vi "Teleop.vi"(10 "Match Info":T1={"Autonomous Elapsed Seconds"=0.0, "TeleOp Elapsed Seconds"=0.0, "Disabled Elapsed Seconds"=0.0, "Visited Autonomous"=FALSE, "Visited TeleOp"=FALSE, "Visited Disabled"=FALSE, "Autonomous Settings"={"Autonomous Style"=enum."Independent", "VI Refnum"=refnum}}, 11 "Call Context":T2) -> ()   [LabVIEW 2016]
doc: "This VI is called for each TeleOp packet received from the DS where the robot is not disabled. It is often used to read from the joysticks and update I/O or to update setpoints for timed control loops. It should complete and return within 20 milliseconds or it may miss DS packets."
uses:
  <vilib>/Rock Robotics/WPI/DriverStation/WPI_DriverStationDerivedRobotMode.ctl
  <vilib>/Rock Robotics/WPI/DriverStation/WPI_DriverStationMatch Info.ctl
  <vilib>/Rock Robotics/WPI/Utilities/WPI_GetSetVariantRefNum.vi
  <vilib>/Rock Robotics/Network Tables/NT Read Boolean.vi
  Robot Global Data.vi
  <vilib>/Rock Robotics/WPI/RobotDrive/WPI_RobotDriveArcadeDrive_Standard(NoSaturation).vi
panel:
  in  "Reset navX":bool
  out "Sample Boolean 0":bool
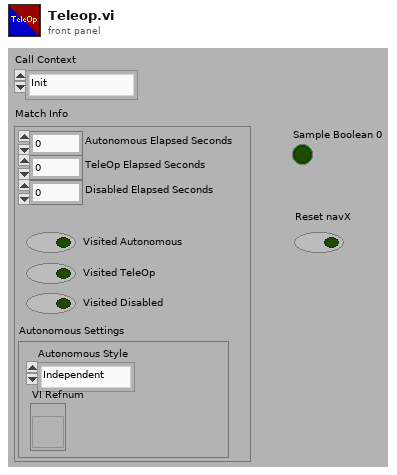
[diagram p1: front panel]
types:
  T1 = typedef "WPI_DriverStationMatch Info.ctl" = cluster{"Autonomous Elapsed Seconds":dbl, "TeleOp Elapsed Seconds":dbl, "Disabled Elapsed Seconds":dbl, "Visited Autonomous":bool, "Visited TeleOp":bool, "Visited Disabled":bool, "Autonomous Settings":cluster{"Autonomous Style":enum16{"Iterative", "Independent"}, "VI Refnum":refnum<vi>}}
  T2 = typedef "WPI_DriverStationDerivedRobotMode.ctl" = enum16{"Init", "Execute", "Stop"}
  T3 = cluster{"Target?":bool, "Angle":dbl, "Distance":dbl}
  T4 = typedef "WPI_RobotDriveDevRef.ctl" = cluster{"DevStatus":errorcluster, "Motors[]":T5[], "Square Inputs":bool, "Max Output":dbl}
  T5 = typedef "WPI_MotorControlDeviceRef.ctl" = cluster{"DeviceStatus":errorcluster, "Type":T6, "PWM":cluster{"PWM Channel":T7, "DeadBand":T8}, "CAN":cluster{"Device Number":u8, "SetOutput VI Ref":variant, "GetOutput VI Ref":variant, "Enable VI Ref":variant, "Disable VI Ref":variant, "Data":variant}, "Invert":bool}
  T6 = typedef "WPI_MotorControlType.ctl" = enum16{"PWM", "CAN"}
  T7 = typedef "FPGA_DIOPWMChannel.ctl" = enum8{"PWM 0", "PWM 1", "PWM 2", "PWM 3", "PWM 4", "PWM 5", "PWM 6", "PWM 7", "PWM 8", "PWM 9", "PWM MXP 0", "PWM MXP 1", "PWM MXP 2", "PWM MXP 3", "PWM MXP 4", "PWM MXP 5", "PWM MXP 6", "PWM MXP 7", "PWM MXP 8", "PWM MXP 9", "Invalid"}
  T8 = typedef "WPI_PWMDeadband.ctl" = cluster{"Name":string, "maxPositivePwm":i32, "minPositivePwm":i32, "centerPwm":i32, "maxNegativePwm":i32, "minNegativePwm":i32, "angularRange":u16}
  T9 = typedef "WPI_JoystickDevRef.ctl" = cluster{"Device":T10}
  T10 = typedef "WPI_JoystickDeviceEnum.ctl" = enum16{"USB 0", "USB 1", "USB 2", "USB 3", "USB 4", "USB 5"}
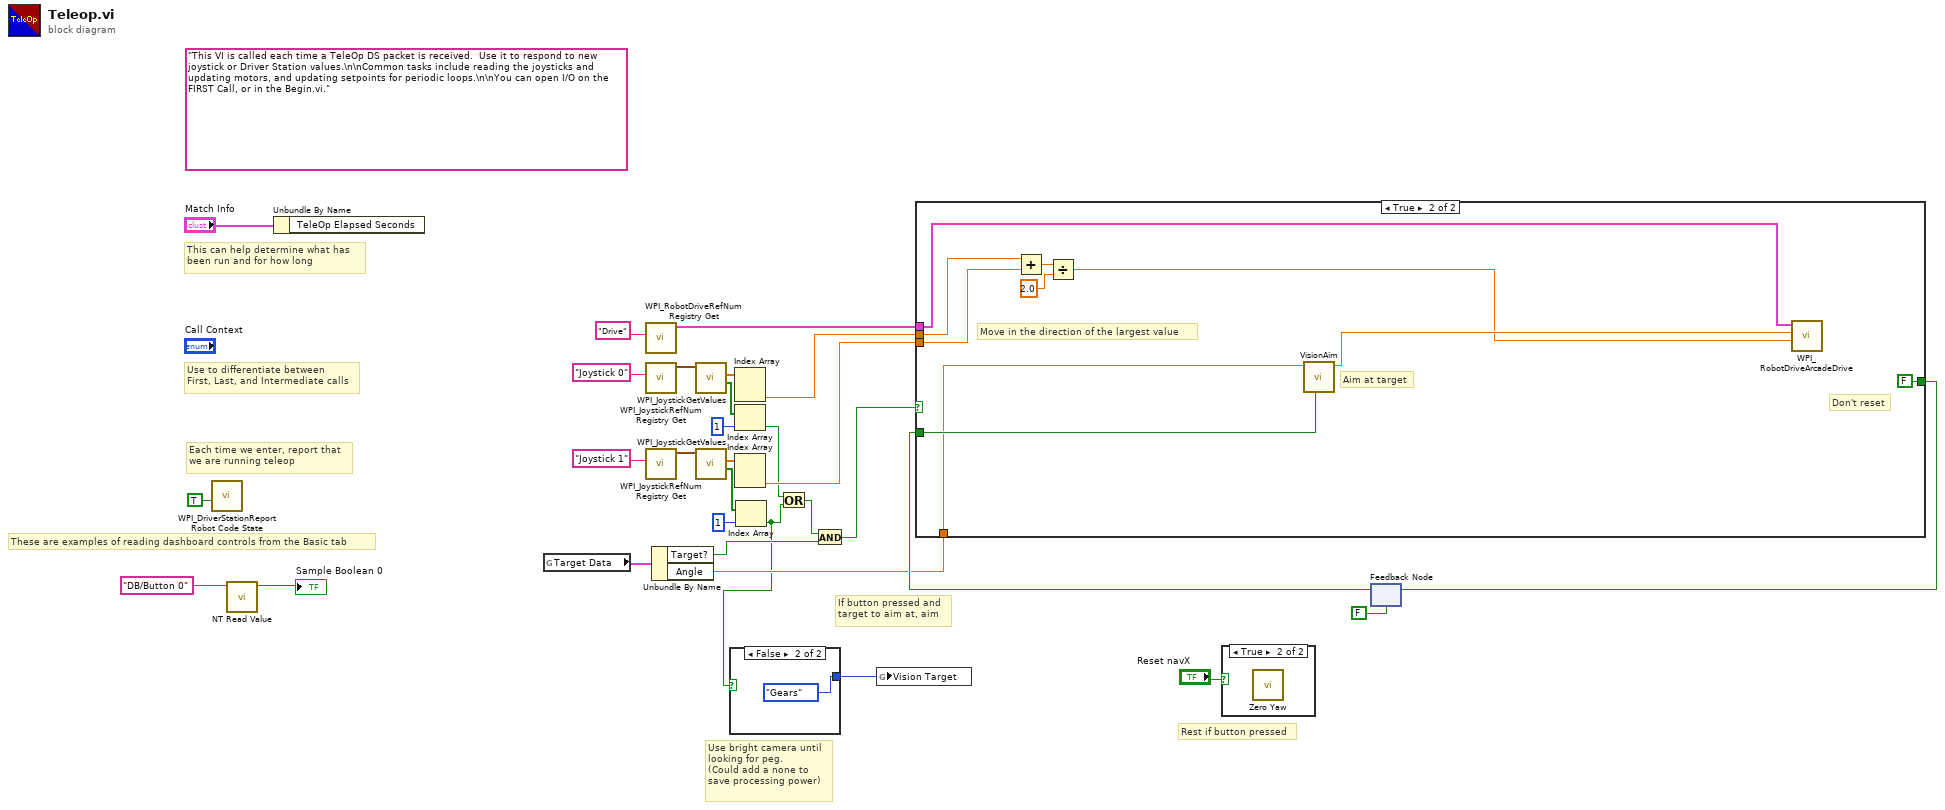
[diagram p0: block diagram]
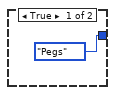
[diagram p2: hidden frame]
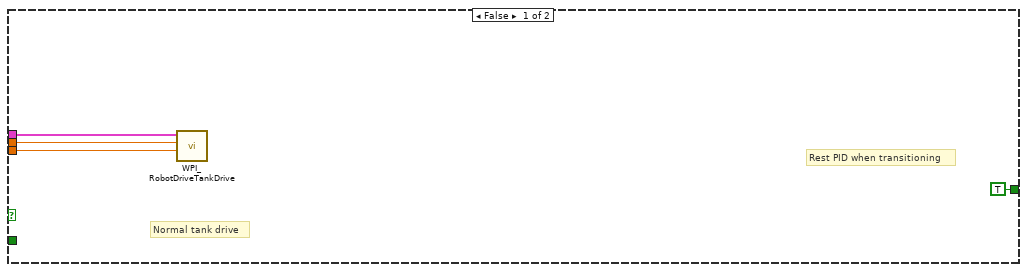
[diagram p4: hidden frame]
diagram:
  (unwired) "This VI is called each time a TeleOp DS packet is received.  Use it to respond to new joystick or Driver Station values.\n\nCommon tasks include reading the joysticks and updating motors, and updating setpoints for periodic loops.\n\nYou can open I/O on the FIRST Call, or in the Begin.vi."
  # "Rest if button pressed"
  # "Use bright camera until\nlooking for peg.\n(Could add a none to\nsave processing power)"
  # "If button pressed and\ntarget to aim at, aim"
  # "These are examples of reading dashboard controls from the Basic tab"
  # "Each time we enter, report that\nwe are running teleop"
  # "Use to differentiate between\nFirst, Last, and Intermediate calls"
  # "This can help determine what has\nbeen run and for how long"
  n1 = call <vilib>:"WPI_DriverStationReport Robot Code State.vi"("TeleOp"=TRUE ("Autonomous")) -> ()  [unwired: 10 in, 1 out]
  n2 = call-poly <vilib>:"NT Read Value.vi"("Name"="DB/Button 0" ("refnum name")) -> ("Boolean"=→"Sample Boolean 0":bool)  [unwired: 9 in, 1 out]
  n3 = Unbundle By Name("Match Info") -> ()  [unwired: 1 out]
  n4 = global read "Robot Global Data.vi" "Target Data"() -> (w6:T3)
  n5 = call <vilib>:"WPI_RobotDriveRefNum Registry Get.vi"("refnum name"="Drive") -> ("RobotDriveDevRef"=w28:T4)  [unwired: 1 in, 9 out]
  n6 = call <vilib>:"WPI_JoystickRefNum Registry Get.vi"("refnum name"="Joystick 0") -> ("JoystickDevRef"=w26:T9)  [unwired: 1 in, 9 out]
  n7 = call <vilib>:"WPI_JoystickRefNum Registry Get.vi"("refnum name"="Joystick 1") -> ("JoystickDevRef"=w20:T9)  [unwired: 1 in, 9 out]
  n8 = Unbundle By Name(w6) -> ("Target?"=w4:bool, "Angle"=w3:dbl)
  n9 = call <vilib>:"WPI_JoystickGetValues.vi"("JoystickDevRef"=w26) -> ("Buttons"=w12:bool[], "Axes"=w22:dbl[])  [unwired: 6 in, 3 out]
  n10 = call <vilib>:"WPI_JoystickGetValues.vi"("JoystickDevRef"=w20) -> ("Buttons"=w16:bool[], "Axes"=w21:dbl[])  [unwired: 6 in, 3 out]
  n11 = Index Array(array=w22) -> (element #2=w17:dbl)  [unwired: 2 in, 1 out]
  n12 = Index Array(array=w12, index=1) -> (element=w11:bool)
  n13 = Index Array(array=w21) -> (element #2=w18:dbl)  [unwired: 2 in, 1 out]
  n14 = Index Array(array=w16, index=1) -> (element=w2:bool)
  n15 = case shown="False" w2 {
    tunnel: [enum16{"Pegs", "Gears"}."Pegs" ("Vision Target") enum16{"Pegs", "Gears"}."Gears" ("Vision Target")] -> w1
    frame True {
    }
    frame False {
    }
  }
  n16 = Or(x=w11, y=w2) -> (x .or. y?=w10:bool)
  n17 = And(x=w10, y=w4) -> (x .and. y?=w14:bool)
  n18 = global write "Robot Global Data.vi" "Vision Target"(w1) -> ()
  n19 = case shown="True" "Reset navX" {
    frame False {
    }
    frame True {
      n20 = call <vilib>:"Zero Yaw.vi"() -> ()  [unwired: 12 in]
    }
  }
  n21 = feedback #1(FALSE ("x .and. y?")) -> (w8:bool)
  n22 = case shown="True" w14 {
    tunnel: w28 -> [w36 w46]
    tunnel: w18 -> [w35 w41]
    tunnel: w17 -> [w34 w40]
    tunnel: w3 -> [_ w43]
    tunnel: [TRUE ("x .and. y?") FALSE ("x .and. y?")] -> w9
    tunnel: w8 -> [_ w44]
    frame False {
      # "Rest PID when transitioning"
      # "Normal tank drive"
      n23 = call <vilib>:"WPI_RobotDriveTankDrive.vi"("Right axis value"=w35, "Left axis value"=w34, "RobotDriveDevRef"=w36) -> ()  [unwired: 6 in, 3 out]
    }
    frame True {
      # "Move in the direction of the largest value"
      # "Aim at target"
      # "Don't reset"
      n24 = Add(x=w40, y=w41) -> (x+y=w39:dbl)
      n25 = Divide(x=w39, y=2.0) -> (x/y=w37:dbl)
      n26 = call "VisionAim.vi"("Reset PID"=w44, "Angle"=w43) -> ("Turn Amount"=w42:dbl)  [unwired: 8 in, 1 out]
      n27 = call-poly <vilib>:"WPI_RobotDriveArcadeDrive.vi"("Y axis value"=w37, "X axis value"=w42, "RobotDriveDevRef"=w46) -> ()  [unwired: 6 in, 3 out]
    }
  }
  n28 = feedback-in #1(w9) -> ()
